vi "TranslatorBooster Is Specifier DataType.vi"(1 "String token":string) -> (0 "Is specifier?":bool)   [LabVIEW 2014, in "Complex Numbers.lvlib"]
uses:
  <vilib>/Aledyne-TSXperts/Arduino Compatible Compiler for LabVIEW/addons/Complex Numbers/Complex Numbers.lvlib
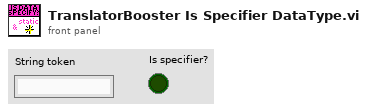
[diagram p1: front panel]
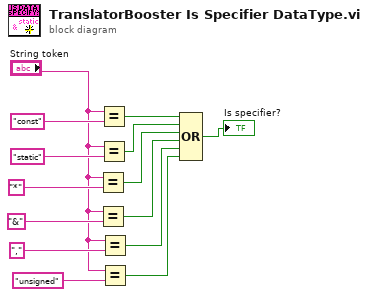
[diagram p0: block diagram]
diagram:
  n1 = Equal?(x="String token", y="*") -> (x = y?=w7:bool)
  n2 = Equal?(x="String token", y="&") -> (x = y?=w6:bool)
  n3 = Equal?(x="String token", y="const") -> (x = y?=w11:bool)
  n4 = Equal?(x="String token", y="static") -> (x = y?=w12:bool)
  n5 = Equal?(x="String token", y=",") -> (x = y?=w3:bool)
  n6 = Equal?(x="String token", y="unsigned") -> (x = y?=w2:bool)
  n7 = Compound Arithmetic op=OR(w11, w12, w7, w6, w3, w2) -> (→"Is specifier?":bool)
